vi "main.vi"() -> ()   [LabVIEW 2015]
uses:
  controls/state.ctl
  controls/timerstate.ctl
panel:
  out "error out":errorcluster
  in  "error in":errorcluster
  in  "App Stop":bool
  in  "Boiler Simulation Controls":T1 {"Flame Sensor Value (%)" scale=0.0..100.0}
  in  "Boiler Controls":T2 {"Fuel Control Valve Position (% Open)" scale=0.0..100.0}
  out "Boiler Status Indicators":T3 {"Time Count (s)" format="%.2f"}
  # "On"
  # "Off"
  # "Closed"
  # "Open"
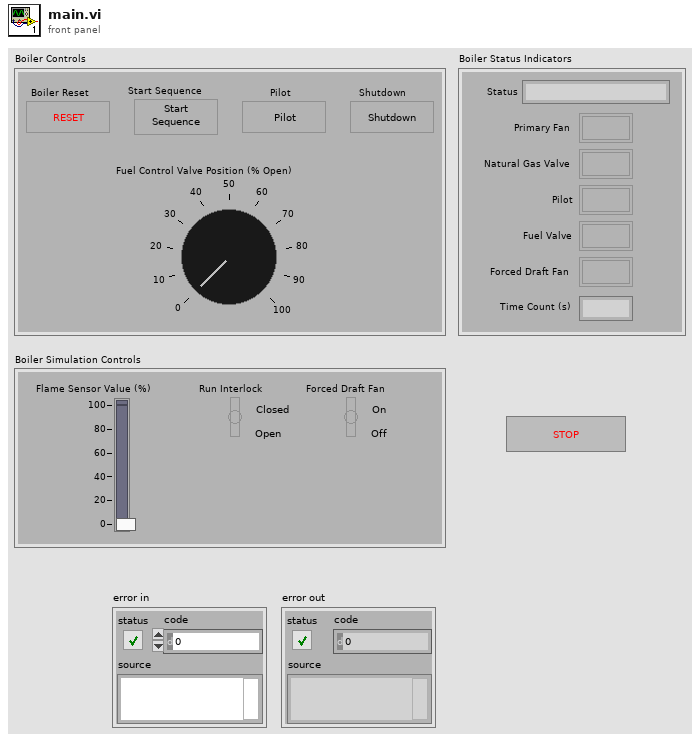
[diagram p1: front panel]
types:
  T1 = cluster{"Flame Sensor Value (%)":dbl, "Run Interlock":bool, "Forced Draft Fan":bool}
  T2 = cluster{"Shutdown":bool, "Pilot Button":bool, "Start Sequence":bool, "Boiler Reset":bool, "Fuel Control Valve Position (% Open)":dbl}
  T3 = cluster{"Time Count (s)":dbl, "Status":string, "Forced Draft Fan":bool, "Fuel Valve":bool, "Pilot Indicator":bool, "Natural Gas Valve":bool, "Primary Fan":bool}
  T4 = typedef "state.ctl" = enum16{"Error", "Exit", "Reset lockout", "Ignition", "Pre Purge Continue", "Pre Purge", "Wait", "Ready", "Initialize", "Purge", "Shutdown", "Run", "Start", "Prove Pilot"}
  T5 = typedef "timerstate.ctl" = enum16{"Stop", "Start"}
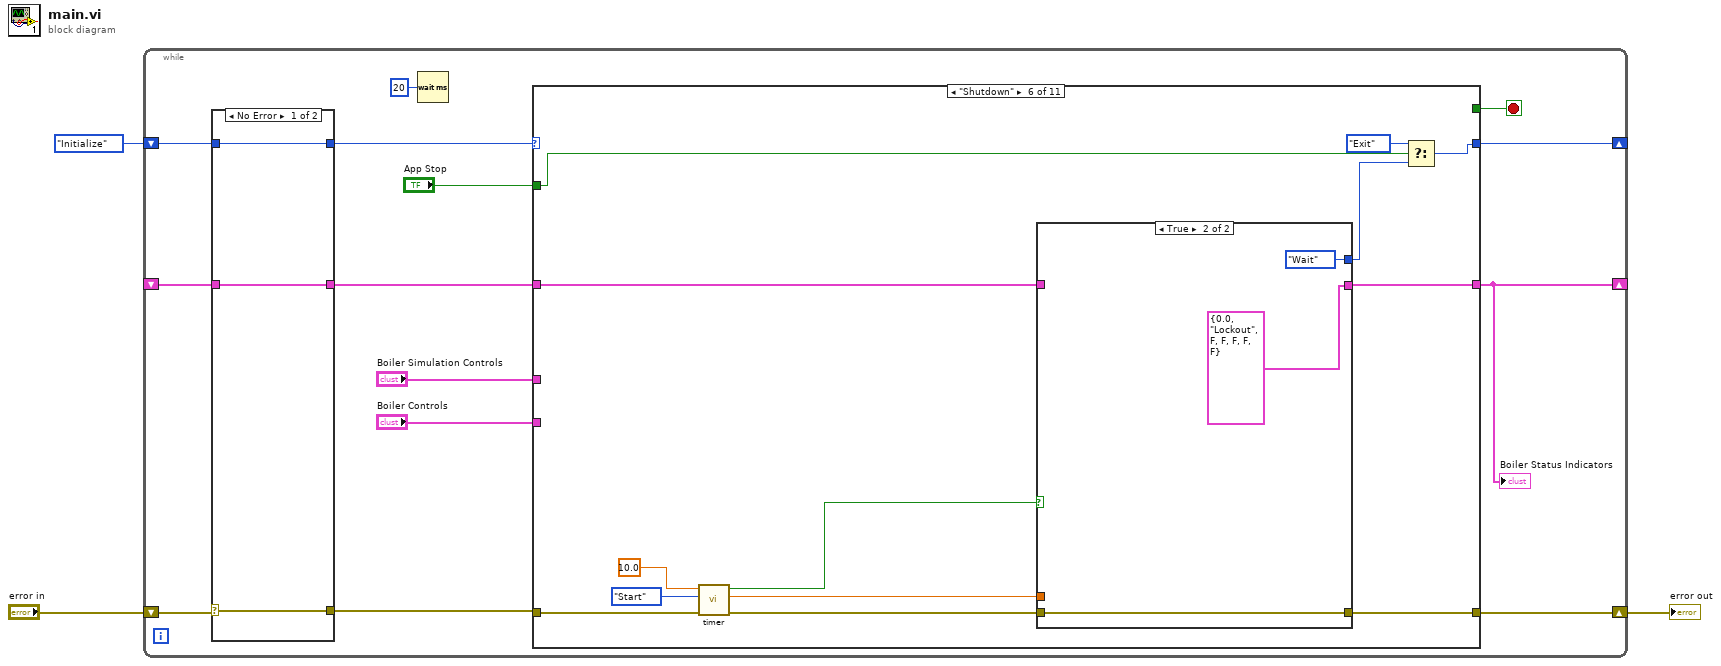
[diagram p0: block diagram]
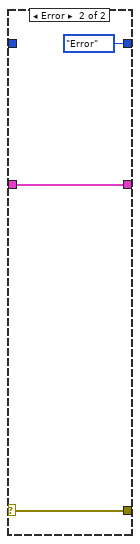
[diagram p2: hidden frame]
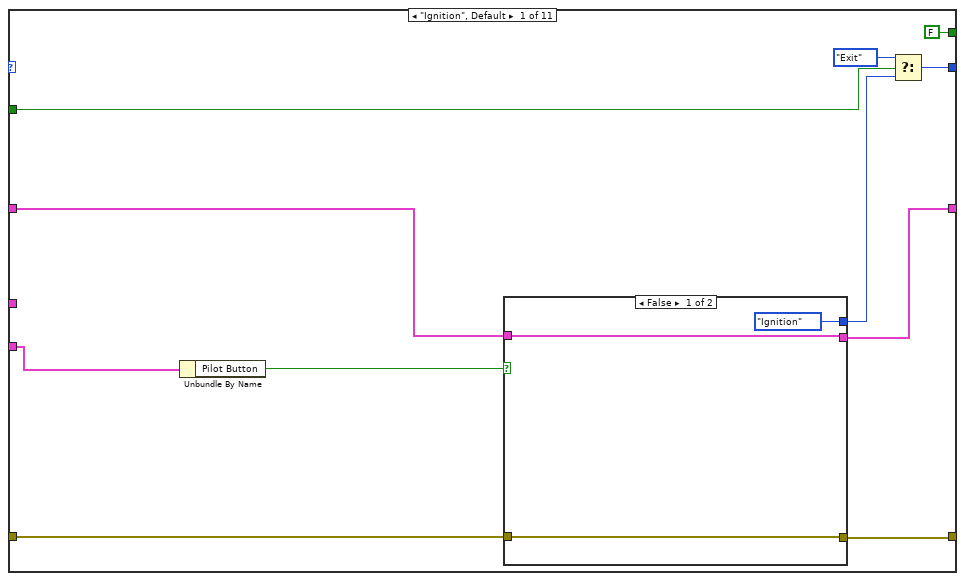
[diagram p3: hidden frame]
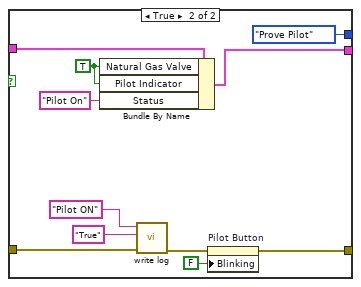
[diagram p4: hidden frame]
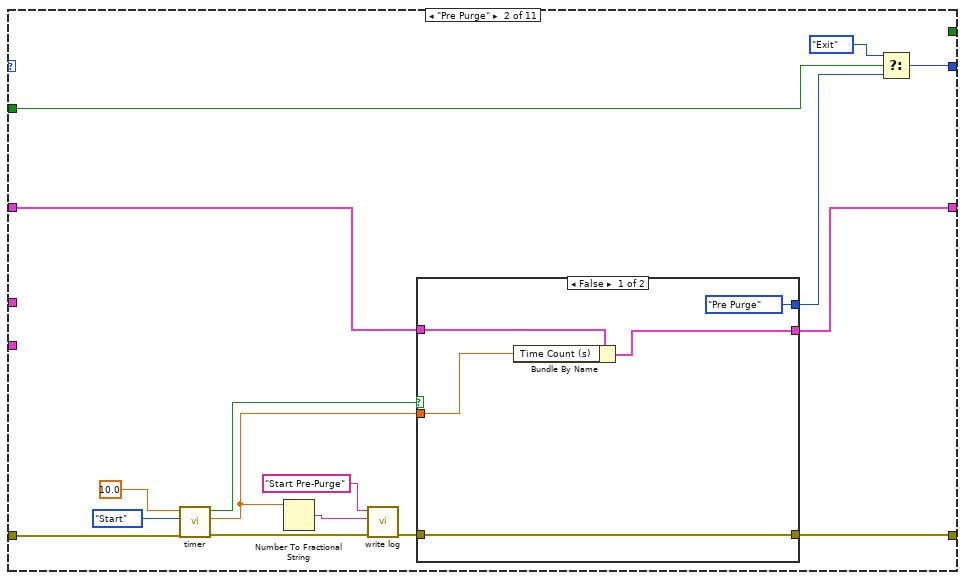
[diagram p5: hidden frame]
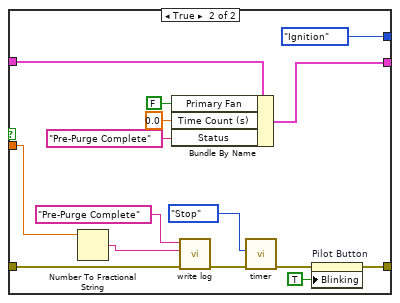
[diagram p6: hidden frame]
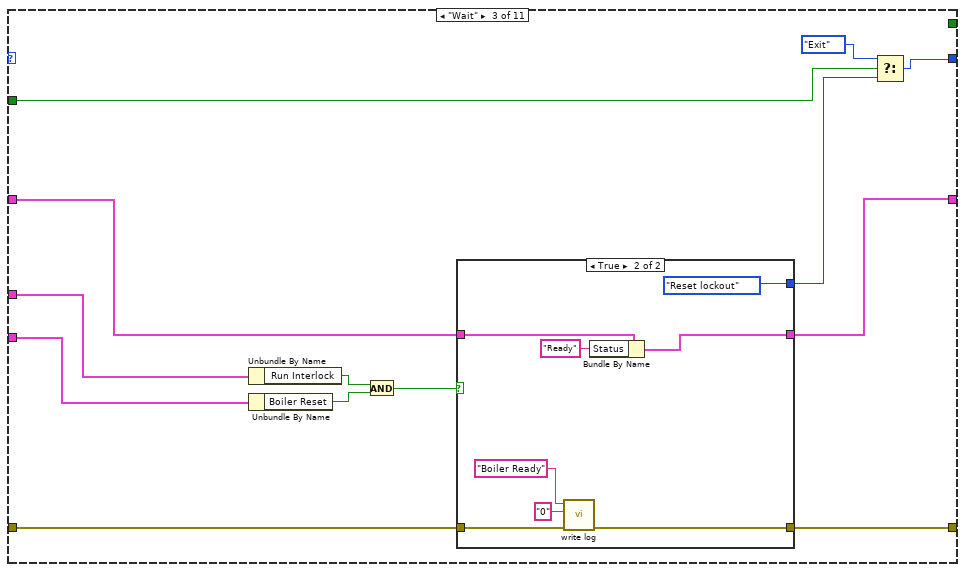
[diagram p7: hidden frame]
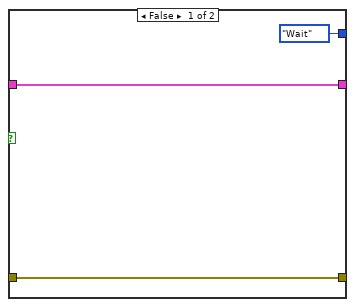
[diagram p8: hidden frame]
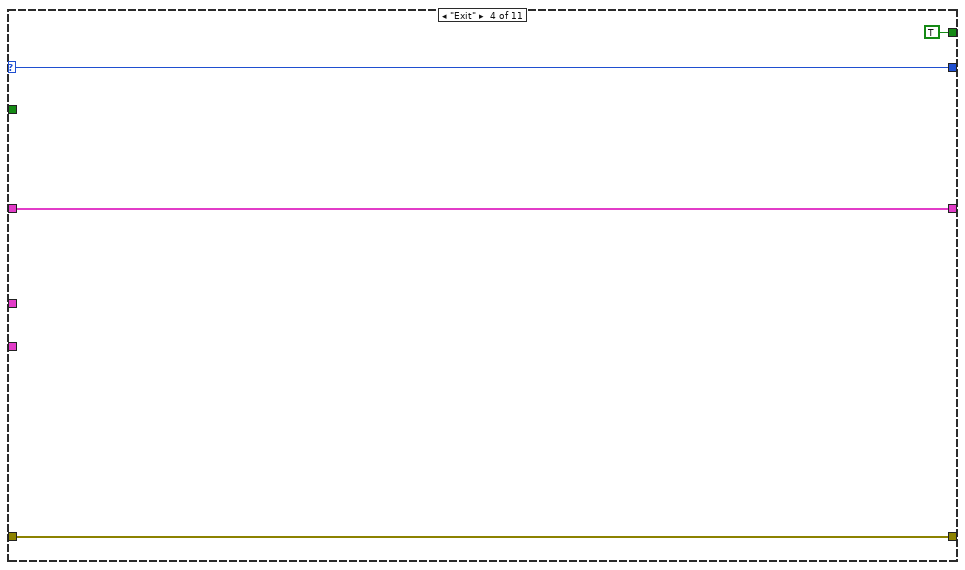
[diagram p9: hidden frame]
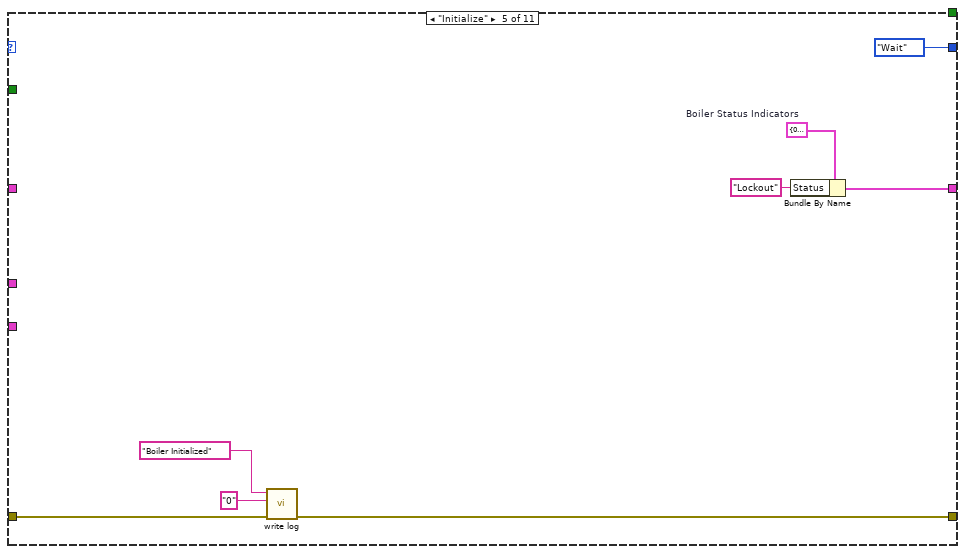
[diagram p10: hidden frame]
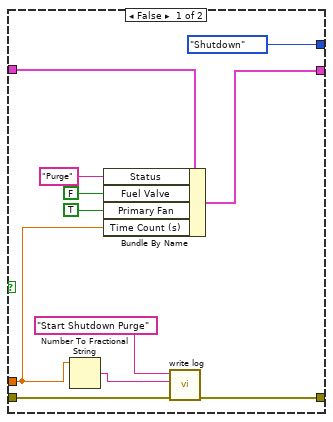
[diagram p11: hidden frame]
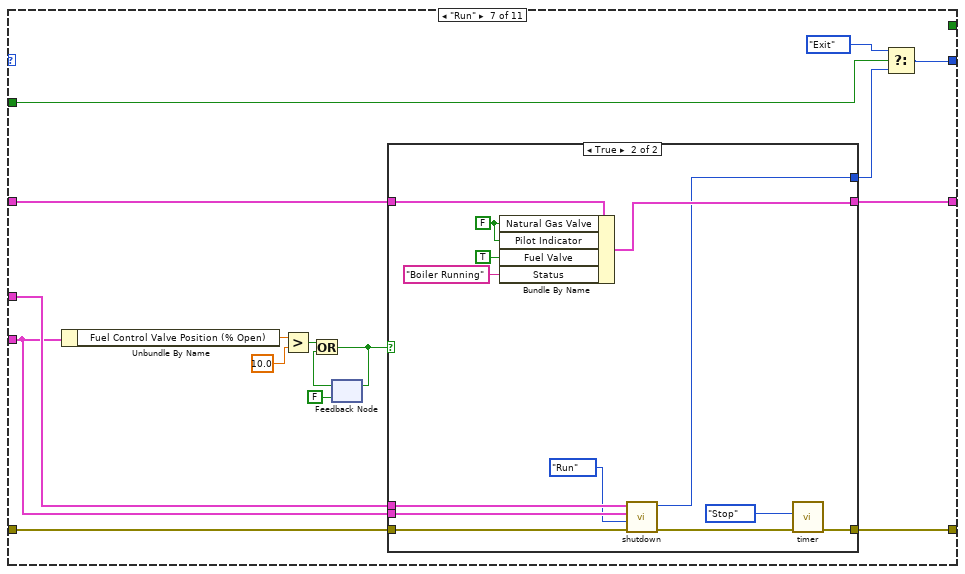
[diagram p12: hidden frame]
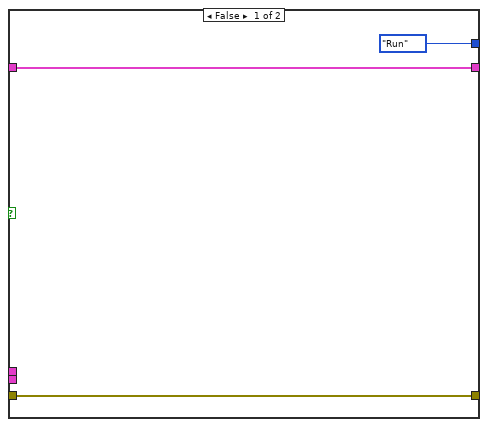
[diagram p13: hidden frame]
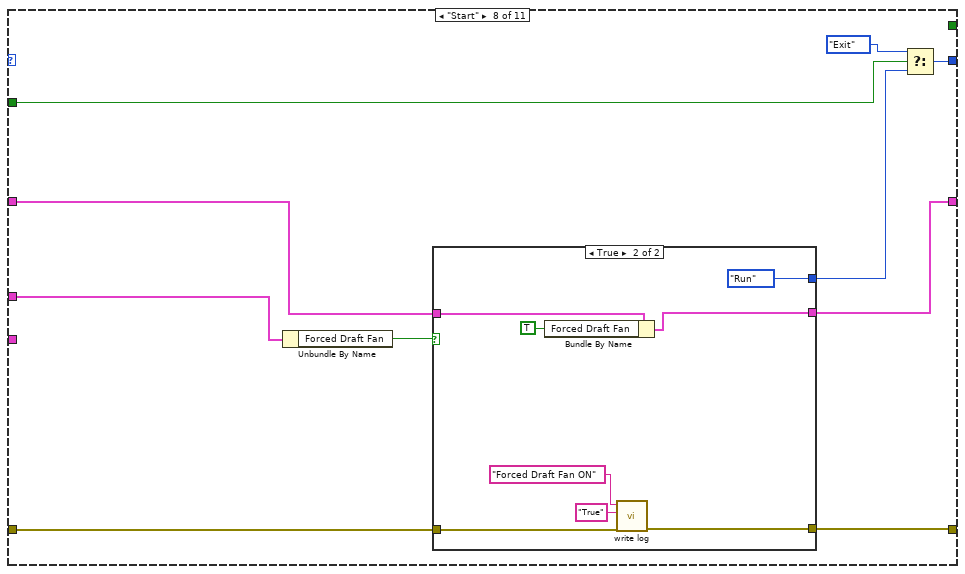
[diagram p14: hidden frame]
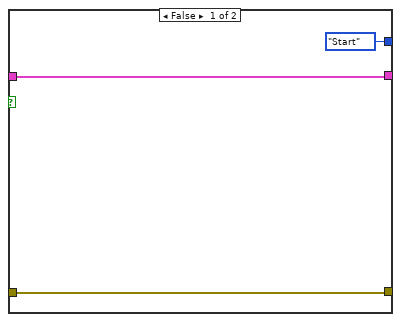
[diagram p15: hidden frame]
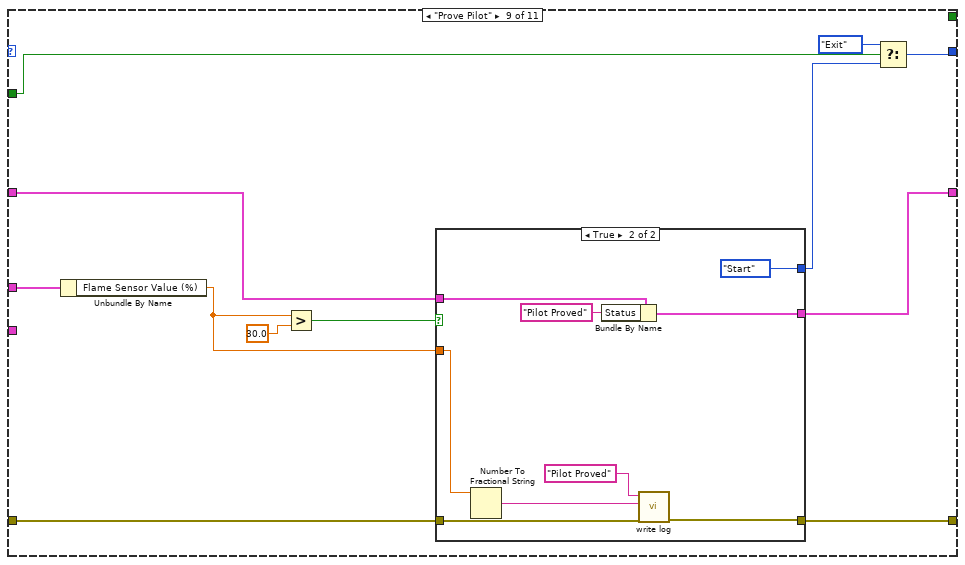
[diagram p16: hidden frame]
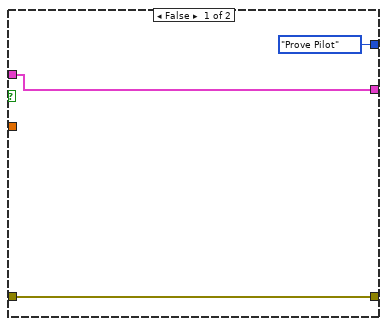
[diagram p17: hidden frame]
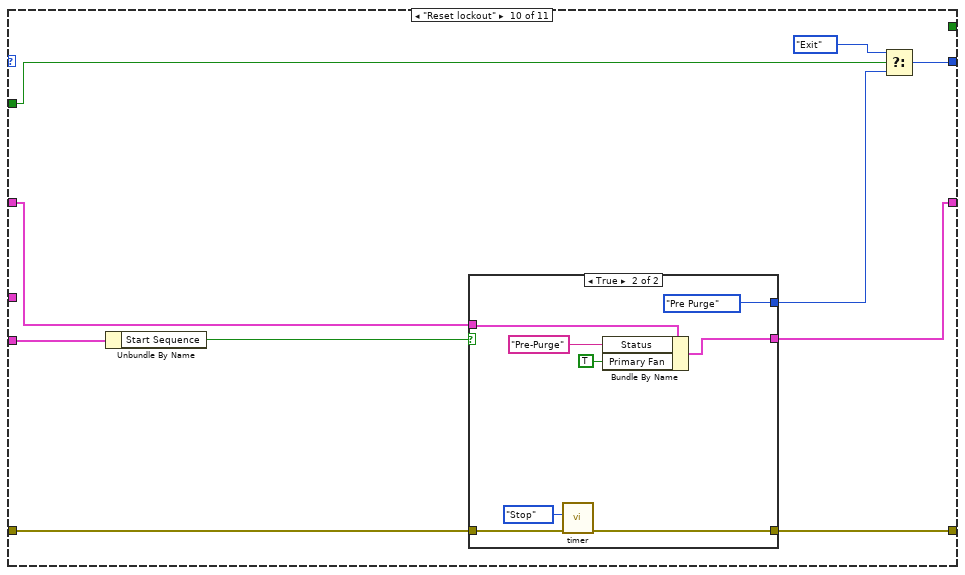
[diagram p18: hidden frame]
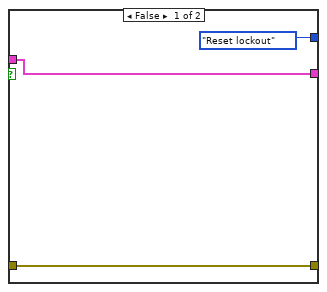
[diagram p19: hidden frame]
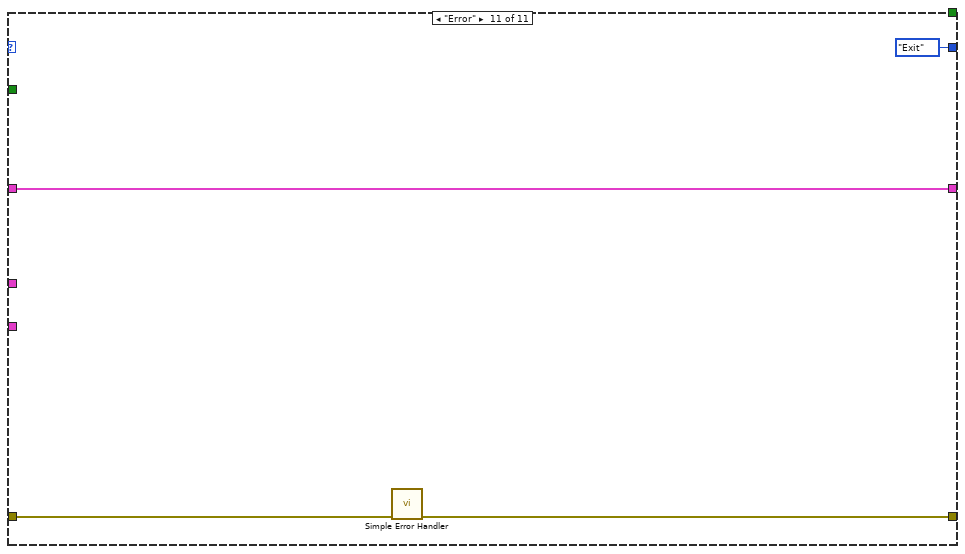
[diagram p20: hidden frame]
diagram:
  n1 = while {
    shift-right: [w16] -> _
    shift-left: _ -> [w6]
    shift-right: [w15] -> _
    shift-left: state."Initialize" ("state") -> [w7]
    shift-right: [w10] -> w1
    shift-left: "error in" -> [w9]
    stop <- w17 stop-if-true
    n2 = case shown="No Error" w9 {
      selector: w9 -> [w18 w22]
      tunnel: [w20 state."Error" ("state")] -> w8
      tunnel: w7 -> [w20 _]
      tunnel: w6 -> [w19 w23]
      tunnel: [w19 w23] -> w5
      tunnel: [w18 w22] -> w4
      frame No Error {
      }
      frame Error {
      }
    }
    n3 = Wait (ms)(milliseconds to wait=u32 20) -> ()  [unwired: 1 out]
    n4 = case shown="\"Shutdown\"" w8 {
      selector: w8 -> [_ _ _ w111 _ _ _ _ _ _ _]
      tunnel: [FALSE _ _ TRUE _ _ _ _ _ _ _] -> w17
      tunnel: w4 -> [w33 w64 w97 w109 w120 w131 w157 w189 w210 w233 w249]
      tunnel: [w30 w53 w91 w109 w119 w129 w152 w186 w203 w234 w248] -> w10
      tunnel: [w28 w57 w86 w110 w116 w125 w156 w184 w206 w225 w247] -> w16
      tunnel: [w24 w49 w88 w111 state."Wait" ("state") w121 w150 w182 w201 w227 state."Exit" ("state")] -> w15
      tunnel: "Boiler Simulation Controls" -> [_ _ w96 _ _ _ w154 w188 w212 _ _]
      tunnel: "Boiler Controls" -> [w32 _ w95 _ _ _ w153 _ _ w232 _]
      tunnel: "App Stop" -> [w27 w51 w90 _ _ w124 w149 w183 w205 w230 _]
      tunnel: w5 -> [w29 w58 w87 w110 _ w126 w155 w185 w207 w226 w247]
      frame "Ignition", Default {
        n5 = Unbundle By Name(w32) -> ("Pilot Button"=w31:bool)
        n6 = case shown="False" w31 {
          tunnel: w33 -> [w35 w48]
          tunnel: [w35 w40] -> w30
          tunnel: w29 -> [w37 w45]
          tunnel: [w37 w39] -> w28
          tunnel: [state."Ignition" ("state") state."Prove Pilot" ("state")] -> w26
          frame False {
          }
          frame True {
            w44 = TRUE ("Natural Gas Valve")
            n7 = Bundle By Name(cluster=w45, "Natural Gas Valve"=w44, "Pilot Indicator"=w44, "Status"="Pilot On") -> (w39:T3)
            n8 = call "write log.vi"("error in (no error)"=w48, "Event data"="True", "Event"="Pilot ON") -> ("error out"=w42:errorcluster)  [unwired: 8 in]
            n9 = property on="Pilot Button" class="Bool"(error in=w42, "Blinking"=FALSE) -> (error out=w40:errorcluster)  [unwired: 1 in, 1 out]
          }
        }
        n10 = Select(t=state."Exit", s=w27, f=w26) -> (s? t:f=w24:T4)
      }
      frame "Pre Purge" {
        n11 = call "timer.vi"("error in"=w64, "timerstate"=timerstate."Start", "limit"=10.0) -> ("error out"=w61:errorcluster, "elapsed"=w55:dbl, "limit out"=w59:bool)  [unwired: 6 in]
        n12 = Number To Fractional String(number=w55) -> (F-format string=w54:string)  [unwired: 3 in]
        n13 = call "write log.vi"("error in (no error)"=w61, "Event data"=w54, "Event"="Start Pre-Purge") -> ("error out"=w60:errorcluster)  [unwired: 8 in]
        n14 = case shown="False" w59 {
          tunnel: w60 -> [w65 w75]
          tunnel: w58 -> [w69 w84]
          tunnel: w55 -> [w68 w72]
          tunnel: [w67 w79] -> w57
          tunnel: [w65 w77] -> w53
          tunnel: [state."Pre Purge" ("state") state."Ignition" ("state")] -> w52
          frame False {
            n15 = Bundle By Name(cluster=w69, "Time Count (s)"=w68) -> (w67:T3)
          }
          frame True {
            n16 = Number To Fractional String(number=w72) -> (F-format string=w71:string)  [unwired: 3 in]
            n17 = Bundle By Name(cluster=w84, "Primary Fan"=FALSE, "Time Count (s)"=0.0, "Status"="Pre-Purge Complete") -> (w79:T3)
            n18 = call "write log.vi"("error in (no error)"=w75, "Event data"=w71, "Event"="Pre-Purge Complete") -> ("error out"=w74:errorcluster)  [unwired: 8 in]
            n19 = call "timer.vi"("error in"=w74, "timerstate"=timerstate."Stop") -> ("error out"=w78:errorcluster)  [unwired: 7 in, 2 out]
            n20 = property on="Pilot Button" class="Bool"(error in=w78, "Blinking"=TRUE) -> (error out=w77:errorcluster)  [unwired: 1 in, 1 out]
          }
        }
        n21 = Select(t=state."Exit", s=w51, f=w52) -> (s? t:f=w49:T4)
      }
      frame "Wait" {
        n22 = Unbundle By Name(w96) -> ("Run Interlock"=w94:bool)
        n23 = Unbundle By Name(w95) -> ("Boiler Reset"=w93:bool)
        n24 = And(x=w94, y=w93) -> (x .and. y?=w92:bool)
        n25 = case shown="True" w92 {
          tunnel: w97 -> [w100 w108]
          tunnel: [w100 w107] -> w91
          tunnel: [state."Wait" ("state") state."Reset lockout" ("state")] -> w89
          tunnel: w87 -> [w98 w103]
          tunnel: [w98 w102] -> w86
          frame False {
          }
          frame True {
            n26 = call "write log.vi"("error in (no error)"=w108, "Event data"="0", "Event"="Boiler Ready") -> ("error out"=w107:errorcluster)  [unwired: 8 in]
            n27 = Bundle By Name(cluster=w103, "Status"="Ready") -> (w102:T3)
          }
        }
        n28 = Select(t=state."Exit", s=w90, f=w89) -> (s? t:f=w88:T4)
      }
      frame "Exit" {
      }
      frame "Initialize" {
        w118 = T3 {"Time Count (s)"=0.0, "Status"="", "Forced Draft Fan"=FALSE, "Fuel Valve"=FALSE, "Pilot Indicator"=FALSE, "Natural Gas Valve"=FALSE, "Primary Fan"=FALSE}  # Boiler Status Indicators
        n29 = call "write log.vi"("error in (no error)"=w120, "Event data"="0", "Event"="Boiler Initialized") -> ("error out"=w119:errorcluster)  [unwired: 8 in]
        n30 = Bundle By Name(cluster=w118, "Status"="Lockout") -> (w116:T3)
      }
      frame "Shutdown" {
        n31 = call "timer.vi"("error in"=w131, "timerstate"=timerstate."Start", "limit"=10.0) -> ("error out"=w130:errorcluster, "elapsed"=w127:dbl, "limit out"=w128:bool)  [unwired: 6 in]
        n32 = case shown="True" w128 {
          tunnel: w130 -> [w144 w145]
          tunnel: [w143 w145] -> w129
          tunnel: w127 -> [w135 _]
          tunnel: w126 -> [w137 _]
          tunnel: [w136 T3 {"Time Count (s)"=0.0, "Status"="Lockout", "Forced Draft Fan"=FALSE, "Fuel Valve"=FALSE, "Pilot Indicator"=FALSE, "Natural Gas Valve"=FALSE, "Primary Fan"=FALSE} ("Boiler Status Indicators")] -> w125
          tunnel: [state."Shutdown" ("state") state."Wait" ("state")] -> w123
          frame False {
            n33 = Number To Fractional String(number=w135) -> (F-format string=w142:string)  [unwired: 3 in]
            n34 = Bundle By Name(cluster=w137, "Status"="Purge", "Fuel Valve"=FALSE, "Primary Fan"=TRUE, "Time Count (s)"=w135) -> (w136:T3)
            n35 = call "write log.vi"("error in (no error)"=w144, "Event data"=w142, "Event"="Start Shutdown Purge") -> ("error out"=w143:errorcluster)  [unwired: 8 in]
          }
          frame True {
          }
        }
        n36 = Select(t=state."Exit", s=w124, f=w123) -> (s? t:f=w121:T4)
      }
      frame "Run" {
        n37 = Unbundle By Name(w153) -> ("Fuel Control Valve Position (% Open)"=w161:dbl)
        n38 = Greater?(x=w161, y=10.0) -> (0:w159:bool)
        n39 = feedback #1(FALSE) -> (w163:bool)
        n40 = Or(x=w159, y=w163) -> (x .or. y?=w158:bool)
        n41 = feedback-in #1(w158) -> ()
        n42 = case shown="True" w158 {
          tunnel: w157 -> [w164 w174]
          tunnel: [w166 w175] -> w156
          tunnel: w155 -> [w166 w179]
          tunnel: [state."Run" ("state") w170] -> w151
          tunnel: w154 -> [_ w173]
          tunnel: w153 -> [_ w172]
          tunnel: [w164 w167] -> w152
          frame False {
          }
          frame True {
            w178 = FALSE ("Natural Gas Valve")
            n43 = Bundle By Name(cluster=w179, "Natural Gas Valve"=w178, "Pilot Indicator"=w178, "Fuel Valve"=TRUE, "Status"="Boiler Running") -> (w175:T3)
            n44 = call "shutdown.vi"("error in"=w174, "state"=state."Run", "Boiler Controls"=w172, "Boiler Simulation Controls"=w173) -> ("error out"=w168:errorcluster, "state out"=w170:T4)  [unwired: 6 in]
            n45 = call "timer.vi"("error in"=w168, "timerstate"=timerstate."Stop") -> ("error out"=w167:errorcluster)  [unwired: 7 in, 2 out]
          }
        }
        n46 = Select(t=state."Exit" ("state"), s=w149, f=w151) -> (s? t:f=w150:T4)
      }
      frame "Start" {
        n47 = Unbundle By Name(w188) -> ("Forced Draft Fan"=w187:bool)
        n48 = case shown="True" w187 {
          tunnel: w189 -> [w191 w200]
          tunnel: [w191 w199] -> w186
          tunnel: w185 -> [w190 w196]
          tunnel: [w190 w194] -> w184
          tunnel: [state."Start" ("state") state."Run" ("state")] -> w180
          frame False {
          }
          frame True {
            n49 = Bundle By Name(cluster=w196, "Forced Draft Fan"=TRUE) -> (w194:T3)
            n50 = call "write log.vi"("error in (no error)"=w200, "Event data"="True", "Event"="Forced Draft Fan ON") -> ("error out"=w199:errorcluster)  [unwired: 8 in]
          }
        }
        n51 = Select(t=state."Exit" ("state"), s=w183, f=w180) -> (s? t:f=w182:T4)
      }
      frame "Prove Pilot" {
        n52 = Unbundle By Name(w212) -> ("Flame Sensor Value (%)"=w208:dbl)
        n53 = Greater?(x=w208, y=30.0) -> (0:w209:bool)
        n54 = case shown="True" w209 {
          tunnel: w210 -> [w214 w223]
          tunnel: w208 -> [_ w224]
          tunnel: w207 -> [w213 w220]
          tunnel: [w213 w218] -> w206
          tunnel: [state."Prove Pilot" ("state") state."Start" ("state")] -> w204
          tunnel: [w214 w216] -> w203
          frame False {
          }
          frame True {
            n55 = Number To Fractional String(number=w224) -> (F-format string=w221:string)  [unwired: 3 in]
            n56 = Bundle By Name(cluster=w220, "Status"="Pilot Proved") -> (w218:T3)
            n57 = call "write log.vi"("error in (no error)"=w223, "Event data"=w221, "Event"="Pilot Proved" ("Event data")) -> ("error out"=w216:errorcluster)  [unwired: 8 in]
          }
        }
        n58 = Select(t=state."Exit", s=w205, f=w204) -> (s? t:f=w201:T4)
      }
      frame "Reset lockout" {
        n59 = Unbundle By Name(w232) -> ("Start Sequence"=w231:bool)
        n60 = case shown="True" w231 {
          tunnel: [w237 w244] -> w234
          tunnel: w233 -> [w237 w245]
          tunnel: [state."Reset lockout" ("state") state."Pre Purge" ("state")] -> w228
          tunnel: w226 -> [w235 w241]
          tunnel: [w235 w239] -> w225
          frame False {
          }
          frame True {
            n61 = call "timer.vi"("error in"=w245, "timerstate"=timerstate."Stop") -> ("error out"=w244:errorcluster)  [unwired: 7 in, 2 out]
            n62 = Bundle By Name(cluster=w241, "Status"="Pre-Purge", "Primary Fan"=TRUE) -> (w239:T3)
          }
        }
        n63 = Select(t=state."Exit" ("state"), s=w230, f=w228) -> (s? t:f=w227:T4)
      }
      frame "Error" {
        n64 = call <vilib>:"Simple Error Handler.vi"("error in (no error)"=w249) -> ("error out"=w248:errorcluster)  [unwired: 4 in, 4 out]
      }
    }
    "Boiler Status Indicators" <- w16
  }
  "error out" <- w1
